vi "Master Setup GetPath(pmgr).vi"(10 "path in":path=path "C:/Revolutionary Engineering/Setup Files/Default/Shop Cell 3/~ETC ECCS Setup Files 06-21-2010 08 56 AM.ect") -> (2 "path array":path[](array[path]))   [LabVIEW 2017]
doc: "Get the path from the *.pmgr"
uses:
  Test Series and Profiles PC/Profile Setup/Profile Setup Controls/Profile Traditional View.ctl
  Test Series and Profiles PC/Profile Setup/Profile Setup Controls/Profile List View.ctl
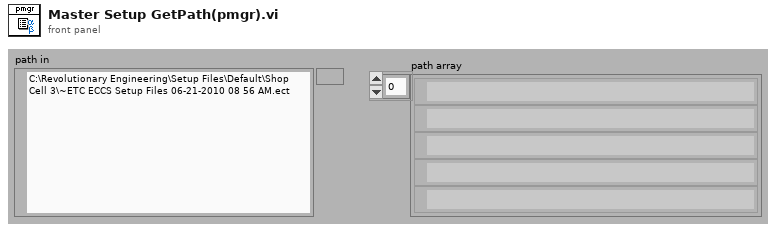
[diagram p1: front panel]
types:
  T1 = enum16{"open", "replace", "create", "open or create", "replace or create", "replace or create with confirmation"}
  T2 = typedef "Profile Traditional View.ctl" = bool
  T3 = typedef "Profile List View.ctl" = bool
  T4 = cluster{"Profile Index":string, "File Path":path, "Link Status":bool, "Traditional View Profile Editor":T2, "List View Profile Editor":T3, "OK Button":bool}[]
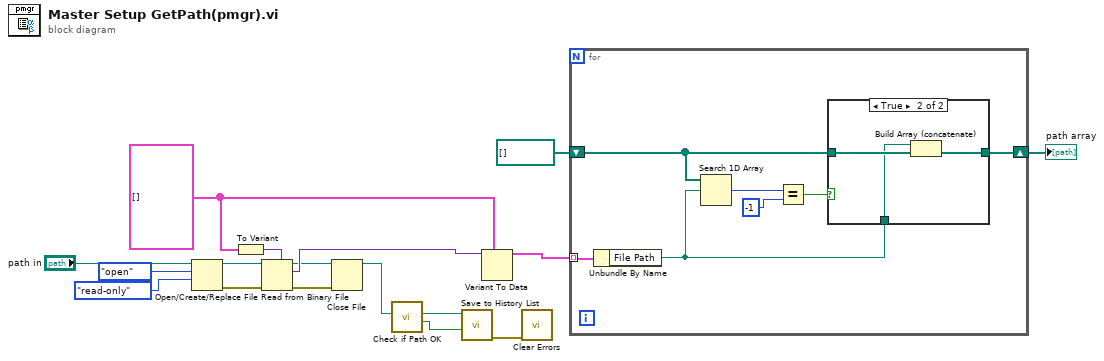
[diagram p0: block diagram]
diagram:
  w11 = T4 []
  n1 = Open/Create/Replace File(file path (use dialog)="path in", operation (0:open)=T1."open", access (0:read/write)=enum16{"read/write", "read-only", "write-only"}."read-only") -> (refnum out=w3:refnum<file>, error out=w2:errorcluster)  [unwired: 3 in, 1 out]
  n2 = To Variant(anything=w11) -> (Variant=w12:variant)
  n3 = Read from Binary File(5:w12, 8:w2, 11:w3) -> (0:w4:errorcluster, 2:w14:variant, 3:w5:refnum<file>)  [unwired: 4 out]
  n4 = Close File(refnum=w5, error in=w4) -> (path=w8:path)  [unwired: 1 out]
  n5 = call "Check if Path OK.vi"("Path"=w8) -> ("Path OK"=w7:bool, "Path"=w9:path)  [unwired: 8 in, 1 out]
  n6 = call "Save to History List.vi"("Write to History File"=w7, "File Path In"=w9) -> ("error out"=w10:errorcluster)  [unwired: 6 in, 3 out]
  n7 = Variant To Data(type=w11, Variant=w14) -> (data=w16:T4)  [unwired: 1 in, 1 out]
  n8 = call <vilib>:"Clear Errors.vi"("error in (no error)"=w10) -> ()  [unwired: 5 in, 2 out]
  n9 = for {
    tunnel: w16 -> [w24] mode=indexing
    shift-right: [w23] -> w15
    shift-left: path[] [] -> [w22]
    n10 = Unbundle By Name(w24) -> ("File Path"=w21:path)
    n11 = Search 1D Array(1D array=w22, element=w21) -> (index of element=w20:i32)  [unwired: 1 in]
    n12 = Equal?(x=w20, y=-1) -> (x = y?=w18:bool)
    n13 = case shown="True" w18 {
      tunnel: [w25 w28] -> w23
      tunnel: w22 -> [w25 w27]
      tunnel: w21 -> [_ w26]
      frame False {
      }
      frame True {
        n14 = Build Array (concatenate)(w26, w27) -> (w28:path[])
      }
    }
  }
  "path array" <- w15
